vi "CM-Read Connector Type.vi"(0 "configuration file path":path=path "C:/PXI Connections.txt", 7 "Device":string="Use BNC-2090", 11 "error in (no error)":errorcluster) -> (4 "file path":path, 8 "Connector Type":T1, 15 "error out":errorcluster)   [LabVIEW 2020]
uses:
  Type Defs/PXISlot XControl/Connector Type.ctl
  Utility VIs/File IO VIs/Configuration File Wrapper VIs/Config-Read Key (string).vi
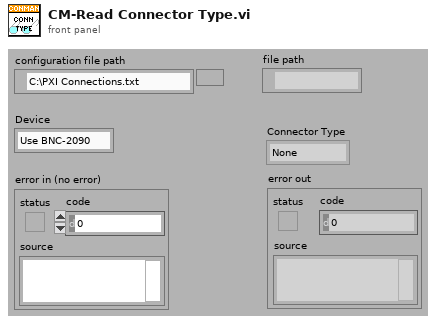
[diagram p1: front panel]
types:
  T1 = typedef "Connector Type.ctl" = enum16{"None", "PXI-4461", "BNC-2110", "BNC-2090", "PXIe-4463", "PXIe-4464"}
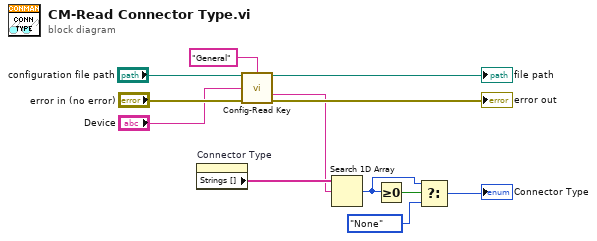
[diagram p0: block diagram]
diagram:
  n1 = property on="Connector Type" class="Enum (strict)"() -> ("Strings []"=w12:string[])  [unwired: 2 in, 2 out]
  n2 = call-poly "Config-Read Key.vi"("configuration file path"="configuration file path", "section"="General", "key"="Device", "error in (no error)"="error in (no error)") -> ("file path"=→"file path":path, "value"=w1:string, "error out"=→"error out":errorcluster)  [unwired: 8 in, 1 out]
  n3 = Search 1D Array(1D array=w12, element=w1) -> (index of element=w8:i32)  [unwired: 1 in]
  n4 = Greater Or Equal To 0?(x=w8) -> (x >= 0?=w11:bool)
  n5 = Select(t=w8, s=w11, f=Connector_Type."None" ("Connector Type")) -> (s? t:f=→"Connector Type":i32)
